vi "Self-Test.vi"(8 "error in (no error)":errorcluster, 11 "NI DMM in":refnum<class "NI DMM.lvclass">) -> (0 "error out":errorcluster, 2 "Result":variant, 3 "NI DMM out":refnum<class "NI DMM.lvclass">)   [LabVIEW 2020, in "NI DMM.lvlib" / "NI DMM.lvclass"]
uses:
  NI DMM.lvclass
  NI DMM.lvclass/NI DMM.ctl
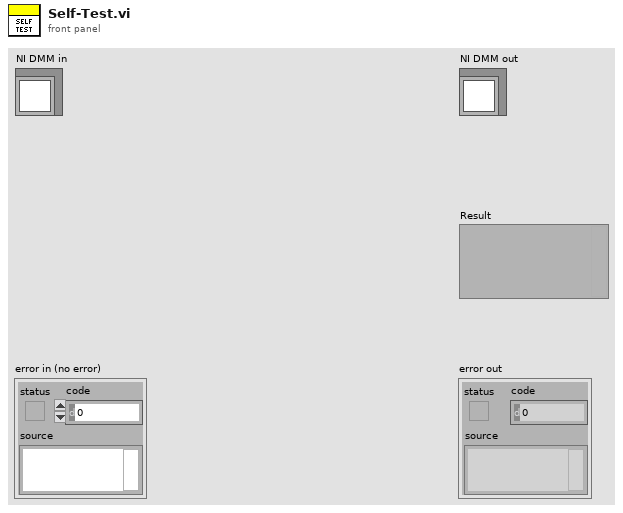
[diagram p1: front panel]
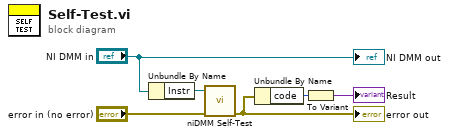
[diagram p0: block diagram]
diagram:
  n1 = Unbundle By Name("NI DMM in") -> ("Instr"=w6:refnum<k15>)
  n2 = call <instrlib>:"niDMM Self-Test.vi"("error in (no error)"="error in (no error)", "instrument handle"=w6) -> ("error out"=w1:errorcluster)  [unwired: 6 in, 3 out]
  "error out" <- w1
  n3 = Unbundle By Name(w1) -> ("code"=w5:i32)
  n4 = To Variant(anything=w5) -> (Variant=→"Result":variant)
  "NI DMM out" <- "NI DMM in"
